vi "Rename Template Plugin Files.vi"(8 "error in":errorcluster, 10 "plugin library path":path, 11 "configuration":T1) -> (0 "error out":errorcluster, 3 "plugin files path":path[](array[path]))   [LabVIEW 2021, in "InstrumentStudio Plug-In Editor.lvlib"]
uses:
  InstrumentStudio Plug-In Editor.lvlib
  Data Holder.ctl
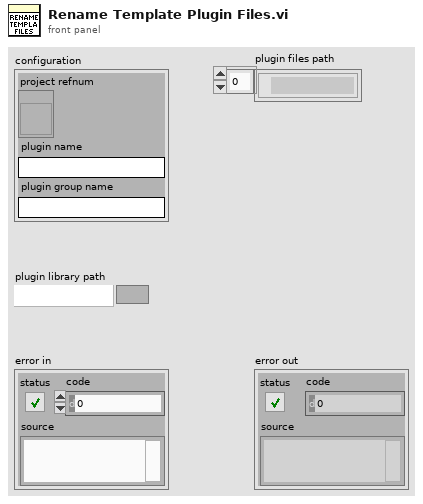
[diagram p1: front panel]
types:
  T1 = typedef "InstrumentStudio Plug-In Editor.lvlib/Data Holder.ctl" = cluster{"project refnum":refnum<vi>, "plugin name":string, "plugin group name":string}
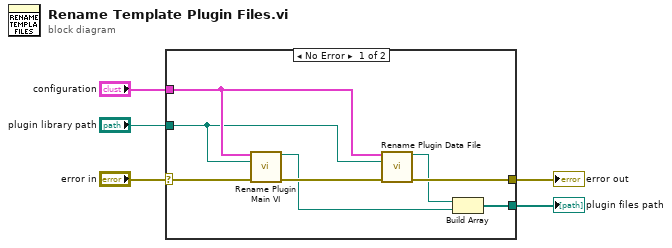
[diagram p0: block diagram]
diagram:
  n1 = case shown="No Error" "error in" {
    selector: "error in" -> [w13 w14]
    tunnel: [w11 w14] -> w2
    tunnel: "configuration" -> [w10 _]
    tunnel: "plugin library path" -> [w6 _]
    tunnel: [w7 _] -> w1
    frame No Error {
      n2 = call "Rename Plugin Main VI.vi"("configuration"=w10, "plugin library path"=w6, "error in"=w13) -> ("plugin main vi path"=w9:path, "error out"=w12:errorcluster)  [unwired: 11 in]
      n3 = call "Rename Plugin Data File.vi"("configuration"=w10, "plugin library path"=w6, "error in"=w12) -> ("plugin data file path"=w8:path, "error out"=w11:errorcluster)  [unwired: 11 in]
      n4 = Build Array(w8, w9) -> (w7:path[])
    }
    frame Error {
    }
  }
  "error out" <- w2
  "plugin files path" <- w1
